vi "proceed.vi"(8 "error in (no error)":errorcluster, 11 "ScanModeDL091001Scaffold in":refnum<class "ImagingModeDL091001Scaffold.lvclass">) -> (0 "error out":errorcluster, 3 "ScanModeDL091001Scaffold out":refnum<class "ImagingModeDL091001Scaffold.lvclass">)   [LabVIEW 2010, in "ImagingModeDL091001Scaffold.lvclass"]
uses:
  ImagingModeDL091001Scaffold.lvclass
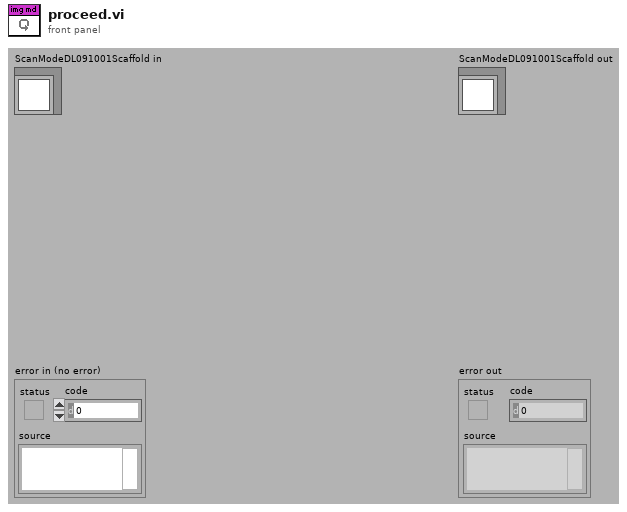
[diagram p1: front panel]
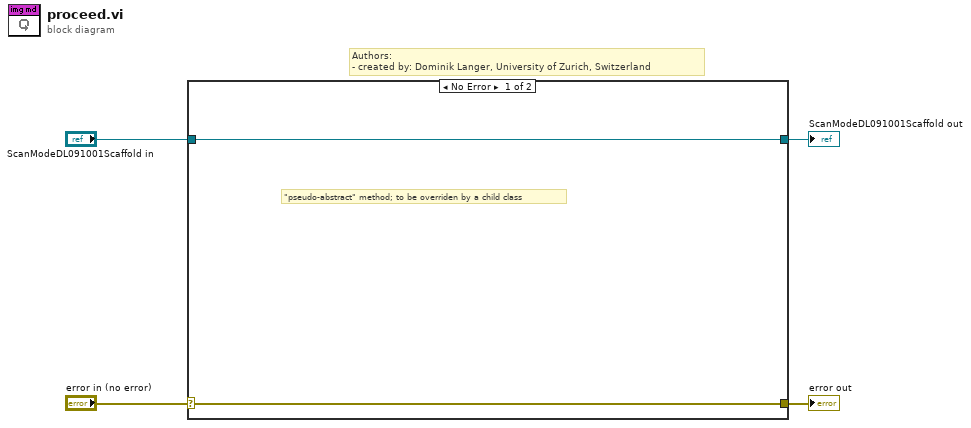
[diagram p0: block diagram]
diagram:
  # "Authors: \n- created by: Dominik Langer, University of Zurich, Switzerland"
  n1 = case shown="No Error" "error in (no error)" {
    selector: "error in (no error)" -> [w5 w8]
    tunnel: [w5 w8] -> w3
    tunnel: [w6 w7] -> w1
    tunnel: "ScanModeDL091001Scaffold in" -> [w6 w7]
    frame No Error {
      # "\"pseudo-abstract\" method; to be overriden by a child class"
    }
    frame Error {
    }
  }
  "error out" <- w3
  "ScanModeDL091001Scaffold out" <- w1
